vi "Add event name.vi"(0 "file path (dialog if empty)":path=path "E:/Daily Lessons/My Experiments and Results/Elcom Dias/Test2.csv", 1 "Event Name":string[](array[string]), 2 "Event Number":u32) -> ()   [LabVIEW 2014]
uses:
  <vilib>/Utility/file.llb/Read From Spreadsheet File (string).vi
  <vilib>/Utility/file.llb/Write To Spreadsheet File (string).vi
panel:
  out "transposed array 2":string[][](array[string])
  out "transposed array":string[][](array[string])
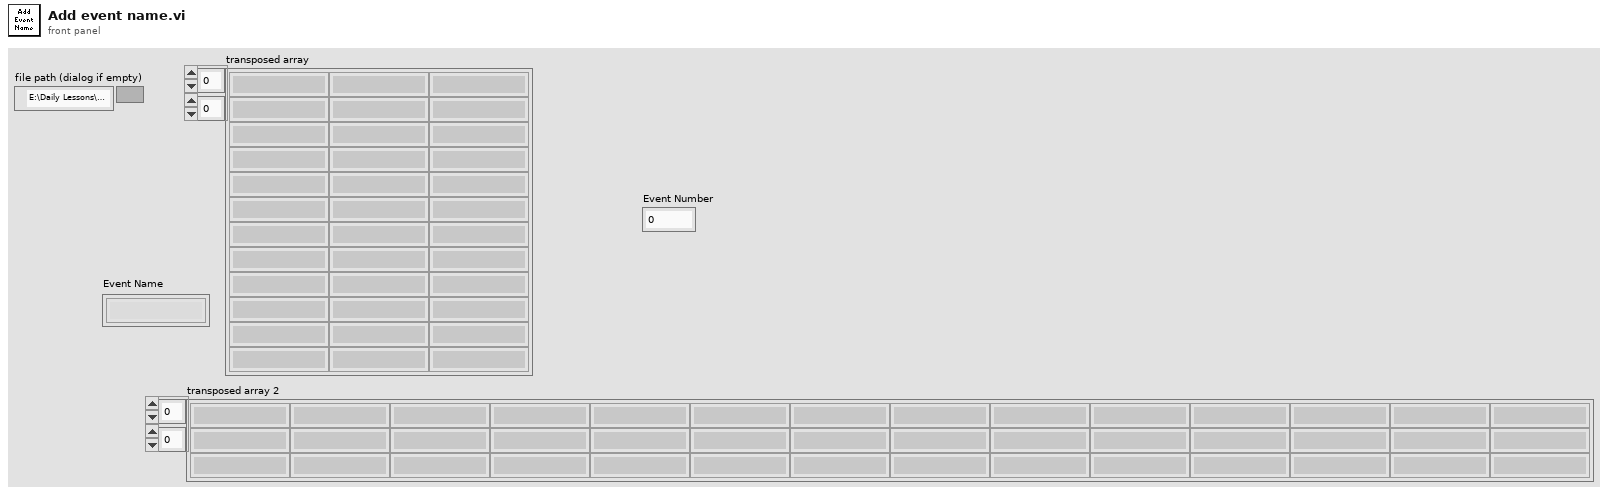
[diagram p1: front panel]
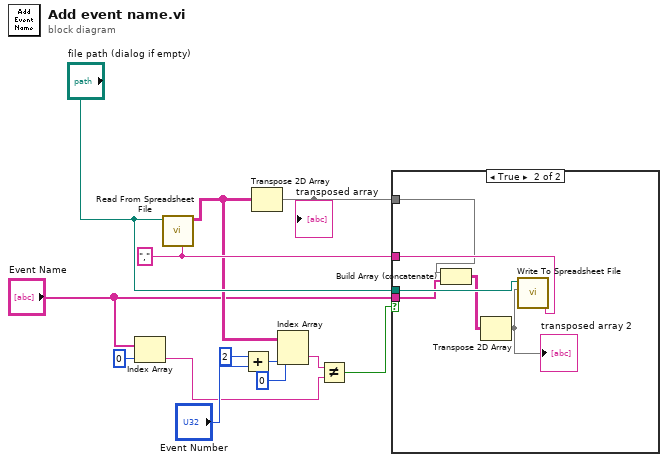
[diagram p0: block diagram]
diagram:
  w12 = "," ("delimiter (\\t)")
  n1 = Index Array(array="Event Name", index=0) -> (element=w2:string)
  n2 = call-poly <vilib>:"Read From Spreadsheet File.vi"("delimiter (\\t)"=w12, "file path (dialog if empty)"="file path (dialog if empty)") -> ("all rows"=w10:string[][])  [unwired: 5 in, 4 out]
  n3 = Add(x=u32 2, y="Event Number") -> (x+y=w9:u32)
  n4 = Transpose 2D Array(2D array=w10) -> (transposed array=w11:string[][])
  "transposed array" <- w11
  n5 = Index Array(array=w10, index (row)=0 ("disabled index (row)"), index (col)=w9) -> (element=w5:string)
  n6 = Not Equal?(x=w5, y=w2) -> (x != y?=w1:bool)
  n7 = case shown="True" w1 {
    tunnel: "file path (dialog if empty)" -> [_ w19]
    tunnel: w12 -> [_ w18]
    tunnel: "Event Name" -> [_ w16]
    tunnel: w11 -> [_ w14]
    frame False {
    }
    frame True {
      n8 = Build Array (concatenate)(w14, w16) -> (w15:string[][])
      n9 = Transpose 2D Array(2D array=w15) -> (transposed array=w17:string[][])
      "transposed array 2" <- w17
      n10 = call-poly <vilib>:"Write To Spreadsheet File.vi"("delimiter (\\t)"=w18, "2D data"=w17, "file path (dialog if empty)"=w19) -> ()  [unwired: 5 in, 1 out]
    }
  }
